vi "Channel.BuildMenuName.vi"(11 "Aliases":T1[](array[typedef])) -> (3 "Aliases Array":string[](array[string]))   [LabVIEW 2013, in "Simple Sequence Tools - Shared.lvlib"]
uses:
  Simple Sequence Tools - Shared.lvlib
  Types/ChannelProperties.ctl
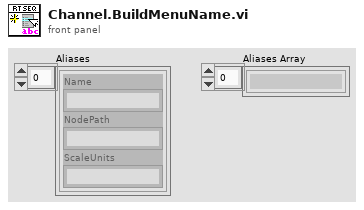
[diagram p1: front panel]
types:
  T1 = typedef "Simple Sequence Tools - Shared.lvlib/ChannelProperties.ctl" = cluster{"Name":string, "NodePath":string, "ScaleUnits":string}
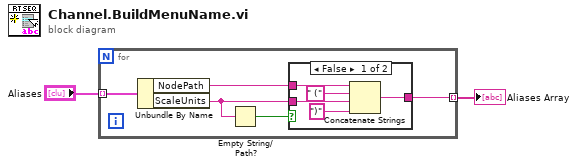
[diagram p0: block diagram]
diagram:
  n1 = for {
    tunnel: "Aliases" -> [w7] mode=indexing
    tunnel: [w5] -> w2 mode=indexing
    n2 = Unbundle By Name(w7) -> ("NodePath"=w6:string, "ScaleUnits"=w4:string)
    n3 = Empty String/Path?(string/path=w4) -> (empty?=w3:bool)
    n4 = case shown="False" w3 {
      tunnel: w6 -> [w10 w13]
      tunnel: [w9 w13] -> w5
      tunnel: w4 -> [w8 _]
      frame False {
        n5 = Concatenate Strings(w10, " (" ("string"), w8, ")" ("string")) -> (w9:string)
      }
      frame True {
      }
    }
  }
  "Aliases Array" <- w2
